vi "H036 Harsh Pandit SCADA Lab 5a Sem 6.vi"() -> ()   [LabVIEW 2018]
panel:
  out "Boolean 9":bool
  out "Boolean 8":bool
  out "Boolean 6":bool
  out "Boolean 5":bool
  out "Boolean 4":bool
  out "Boolean 2":bool
  out "Boolean":bool
  # "Experiment 5a: Create a VI to display 0 to 9 sequentially on 7 segment display using sequence\nstructure"
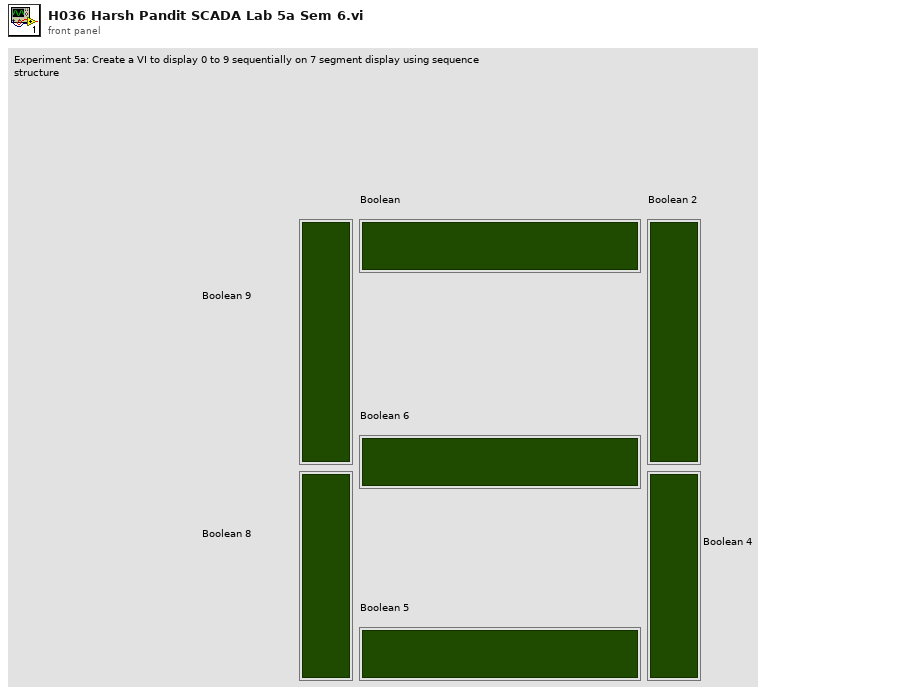
[diagram p1: front panel]
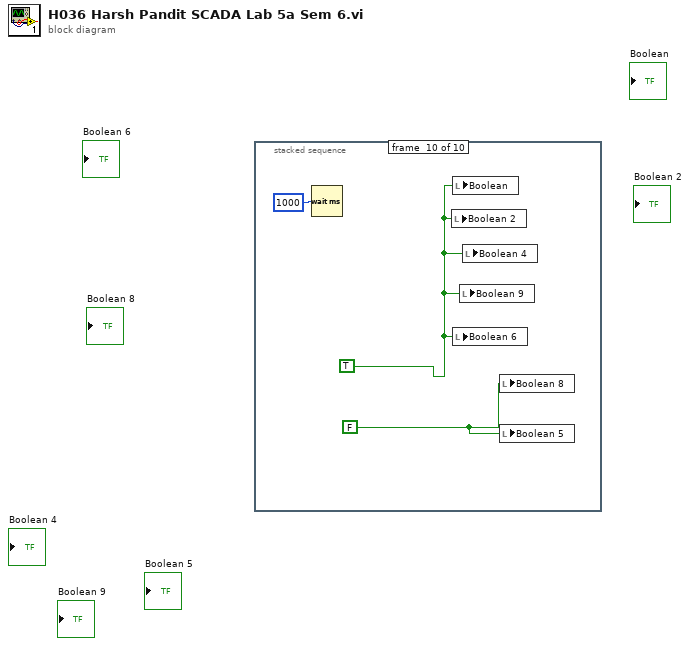
[diagram p0: block diagram]
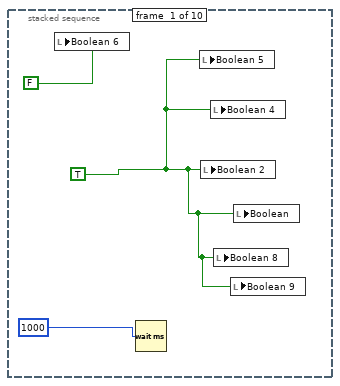
[diagram p2: hidden frame]
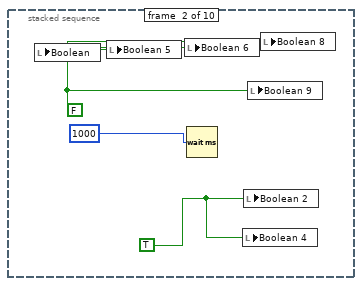
[diagram p3: hidden frame]
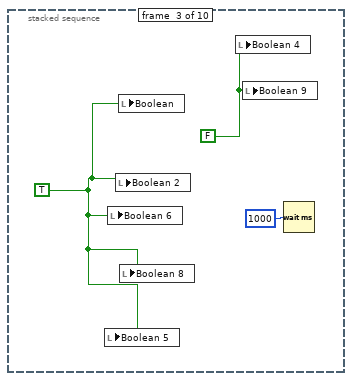
[diagram p4: hidden frame]
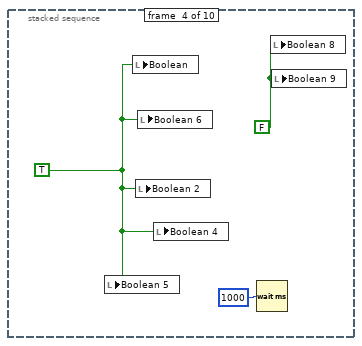
[diagram p5: hidden frame]
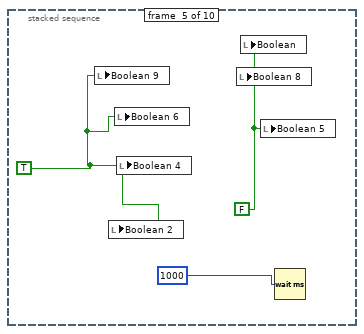
[diagram p6: hidden frame]
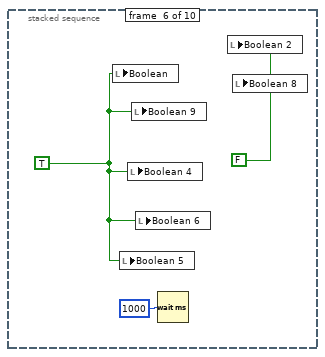
[diagram p7: hidden frame]
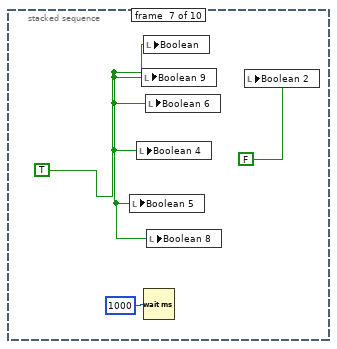
[diagram p8: hidden frame]
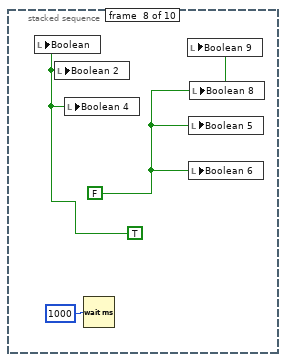
[diagram p9: hidden frame]
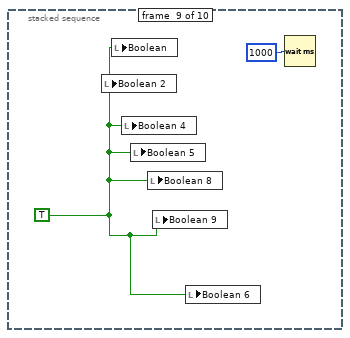
[diagram p10: hidden frame]
diagram:
  n1 = stacked-sequence {
    frame #0 {
      w1 = TRUE
      n2 = local write "Boolean 6"(FALSE) -> ()
      n3 = Wait (ms)(milliseconds to wait=1000) -> ()  [unwired: 1 out]
      n4 = local write "Boolean 5"(w1) -> ()
      n5 = local write "Boolean 2"(w1) -> ()
      n6 = local write "Boolean 4"(w1) -> ()
      n7 = local write "Boolean 8"(w1) -> ()
      n8 = local write "Boolean 9"(w1) -> ()
      n9 = local write "Boolean"(w1) -> ()
    }
    frame #1 {
      w4 = TRUE
      w6 = FALSE
      n10 = local write "Boolean"(w6) -> ()
      n11 = local write "Boolean 5"(w6) -> ()
      n12 = local write "Boolean 6"(w6) -> ()
      n13 = Wait (ms)(milliseconds to wait=1000) -> ()  [unwired: 1 out]
      n14 = local write "Boolean 4"(w4) -> ()
      n15 = local write "Boolean 2"(w4) -> ()
      n16 = local write "Boolean 9"(w6) -> ()
      n17 = local write "Boolean 8"(w6) -> ()
    }
    frame #2 {
      w7 = TRUE
      w9 = FALSE
      n18 = local write "Boolean 5"(w7) -> ()
      n19 = local write "Boolean 6"(w7) -> ()
      n20 = local write "Boolean 2"(w7) -> ()
      n21 = local write "Boolean"(w7) -> ()
      n22 = local write "Boolean 8"(w7) -> ()
      n23 = local write "Boolean 4"(w9) -> ()
      n24 = local write "Boolean 9"(w9) -> ()
      n25 = Wait (ms)(milliseconds to wait=1000) -> ()  [unwired: 1 out]
    }
    frame #3 {
      w10 = TRUE
      w12 = FALSE
      n26 = local write "Boolean 5"(w10) -> ()
      n27 = local write "Boolean"(w10) -> ()
      n28 = local write "Boolean 2"(w10) -> ()
      n29 = local write "Boolean 6"(w10) -> ()
      n30 = local write "Boolean 4"(w10) -> ()
      n31 = Wait (ms)(milliseconds to wait=1000) -> ()  [unwired: 1 out]
      n32 = local write "Boolean 8"(w12) -> ()
      n33 = local write "Boolean 9"(w12) -> ()
    }
    frame #4 {
      w13 = TRUE
      w15 = FALSE
      n34 = local write "Boolean 9"(w13) -> ()
      n35 = local write "Boolean 2"(w13) -> ()
      n36 = local write "Boolean 6"(w13) -> ()
      n37 = local write "Boolean 4"(w13) -> ()
      n38 = local write "Boolean 8"(w15) -> ()
      n39 = local write "Boolean"(w15) -> ()
      n40 = local write "Boolean 5"(w15) -> ()
      n41 = Wait (ms)(milliseconds to wait=1000) -> ()  [unwired: 1 out]
    }
    frame #5 {
      w16 = TRUE
      w18 = FALSE
      n42 = local write "Boolean"(w16) -> ()
      n43 = local write "Boolean 5"(w16) -> ()
      n44 = local write "Boolean 4"(w16) -> ()
      n45 = local write "Boolean 9"(w16) -> ()
      n46 = local write "Boolean 6"(w16) -> ()
      n47 = Wait (ms)(milliseconds to wait=1000) -> ()  [unwired: 1 out]
      n48 = local write "Boolean 2"(w18) -> ()
      n49 = local write "Boolean 8"(w18) -> ()
    }
    frame #6 {
      w19 = TRUE
      n50 = local write "Boolean 5"(w19) -> ()
      n51 = local write "Boolean 4"(w19) -> ()
      n52 = local write "Boolean 9"(w19) -> ()
      n53 = local write "Boolean"(w19) -> ()
      n54 = Wait (ms)(milliseconds to wait=1000) -> ()  [unwired: 1 out]
      n55 = local write "Boolean 6"(w19) -> ()
      n56 = local write "Boolean 8"(w19) -> ()
      n57 = local write "Boolean 2"(FALSE) -> ()
    }
    frame #7 {
      w22 = TRUE
      w24 = FALSE
      n58 = local write "Boolean"(w22) -> ()
      n59 = local write "Boolean 2"(w22) -> ()
      n60 = local write "Boolean 4"(w22) -> ()
      n61 = Wait (ms)(milliseconds to wait=1000) -> ()  [unwired: 1 out]
      n62 = local write "Boolean 9"(w24) -> ()
      n63 = local write "Boolean 5"(w24) -> ()
      n64 = local write "Boolean 6"(w24) -> ()
      n65 = local write "Boolean 8"(w24) -> ()
    }
    frame #8 {
      w25 = TRUE
      n66 = local write "Boolean 2"(w25) -> ()
      n67 = local write "Boolean"(w25) -> ()
      n68 = local write "Boolean 4"(w25) -> ()
      n69 = local write "Boolean 5"(w25) -> ()
      n70 = local write "Boolean 8"(w25) -> ()
      n71 = local write "Boolean 9"(w25) -> ()
      n72 = local write "Boolean 6"(w25) -> ()
      n73 = Wait (ms)(milliseconds to wait=1000) -> ()  [unwired: 1 out]
    }
    frame #9 {
      w27 = TRUE
      w29 = FALSE
      n74 = Wait (ms)(milliseconds to wait=1000) -> ()  [unwired: 1 out]
      n75 = local write "Boolean 2"(w27) -> ()
      n76 = local write "Boolean"(w27) -> ()
      n77 = local write "Boolean 6"(w27) -> ()
      n78 = local write "Boolean 9"(w27) -> ()
      n79 = local write "Boolean 4"(w27) -> ()
      n80 = local write "Boolean 8"(w29) -> ()
      n81 = local write "Boolean 5"(w29) -> ()
    }
  }
